vi "Save Report Information.vi"(8 "error in (no error)":errorcluster, 10 "Report Information.lvclass":refnum<class "Report Information.lvclass">, 11 "TestMonitor in":refnum<class "TestMonitor.lvclass">) -> (0 "error out":errorcluster, 3 "TestMonitor out":refnum<class "TestMonitor.lvclass">)   [LabVIEW 2018, in "TestMonitor.lvclass"]
doc: "This VI will take the Report Information, format it and write it to the permanent report."
uses:
  TestMonitor.lvclass
  Report Information/Report Information.lvclass
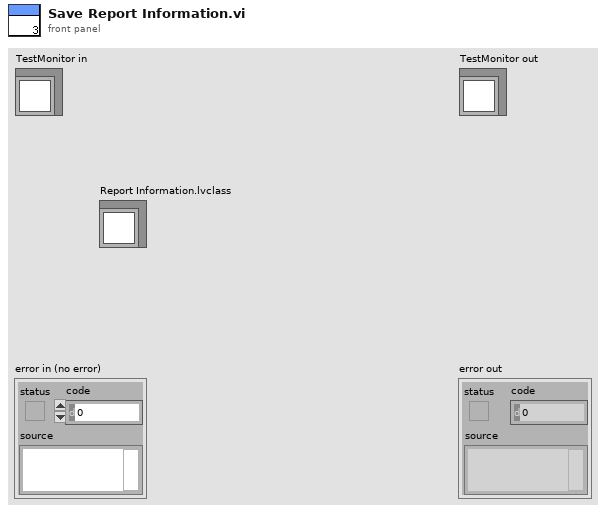
[diagram p1: front panel]
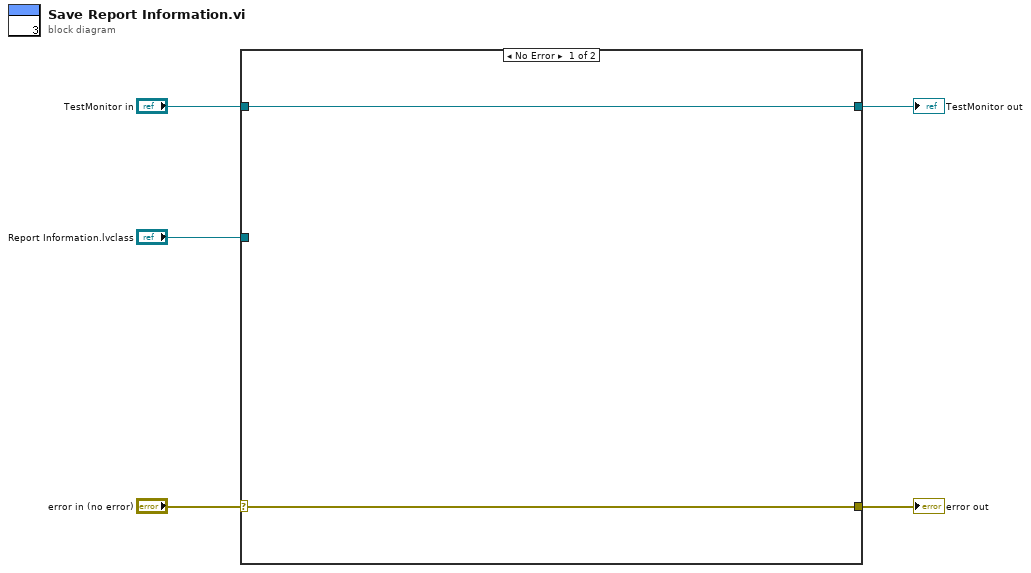
[diagram p0: block diagram]
diagram:
  n1 = case shown="No Error" "error in (no error)" {
    selector: "error in (no error)" -> [w7 _]
    tunnel: [w7 _] -> w5
    tunnel: [w6 w8] -> w3
    tunnel: "TestMonitor in" -> [w6 w8]
    tunnel: "Report Information.lvclass" -> [_ _]
    frame No Error {
    }
    frame Error {
    }
  }
  "error out" <- w5
  "TestMonitor out" <- w3
